vi "my diraction.vi"(7 "?":T2[](array[typedef]), 8 "Empty Directions":T1[](array[typedef]), 9 "my diraction":T1, 10 "curve_rate":dbl) -> (0 "you may act":bool, 1 "Direction for act":i16, 3 "Direction":T1)   [LabVIEW 2020, in "The_Hill_Youth.lvlib" / "MySquare.lvclass"]
uses:
  MySquare.lvclass
  SquareBattle/Direction.ctl
  MyTeam/map_point.ctl
  SquareBattle/SquareBattle.lvlib
panel:
  out "32bit integer":i32
  out "Waveform Chart":dbl(graph)
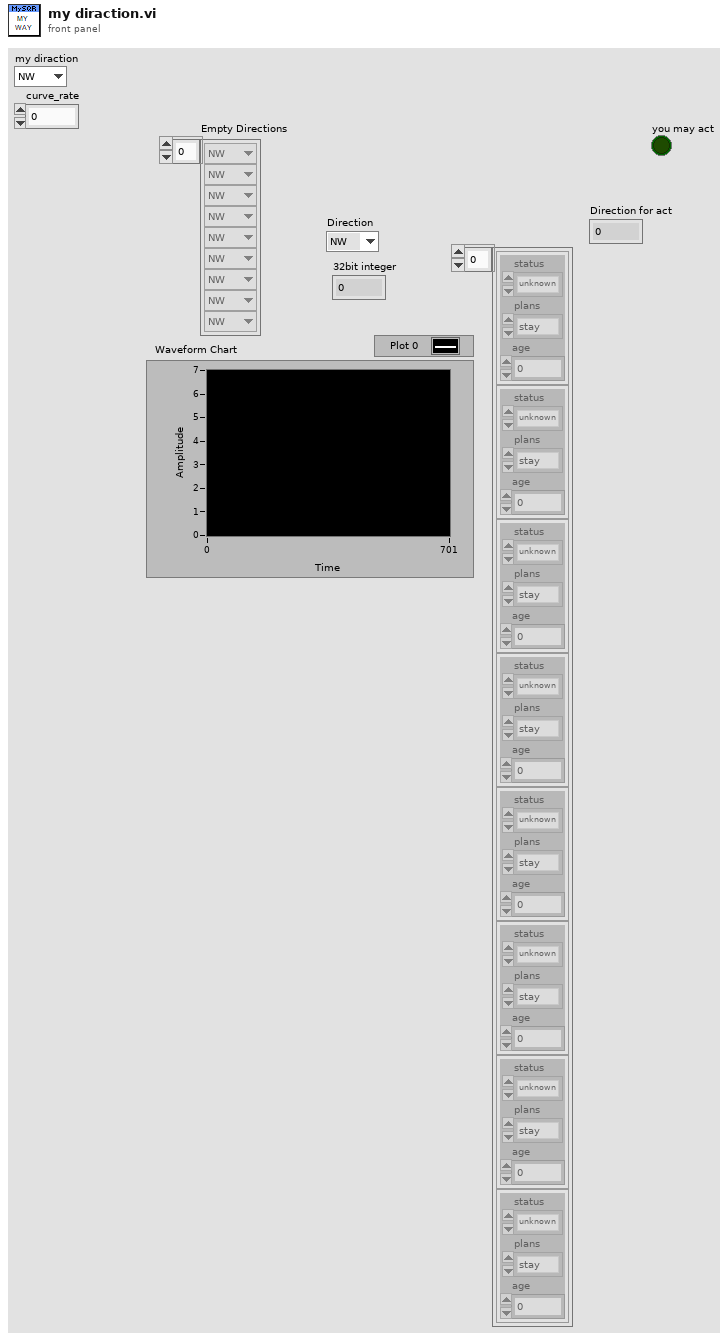
[diagram p1: front panel]
types:
  T1 = typedef "SquareBattle.lvlib/Direction.ctl" = enum16{"NW", "N", "NE", "E", "SE", "S", "SW", "W"}
  T2 = typedef "map_point.ctl" = cluster{"status":enum16{"unknown", "frind", "enemy", "empty"}, "plans":enum16{"stay", "duplicate", "attack", "move to", "no plans"}, "age":dbl}
  T3 = enum16{"stay", "duplicate", "attack", "move to", "no plans"}
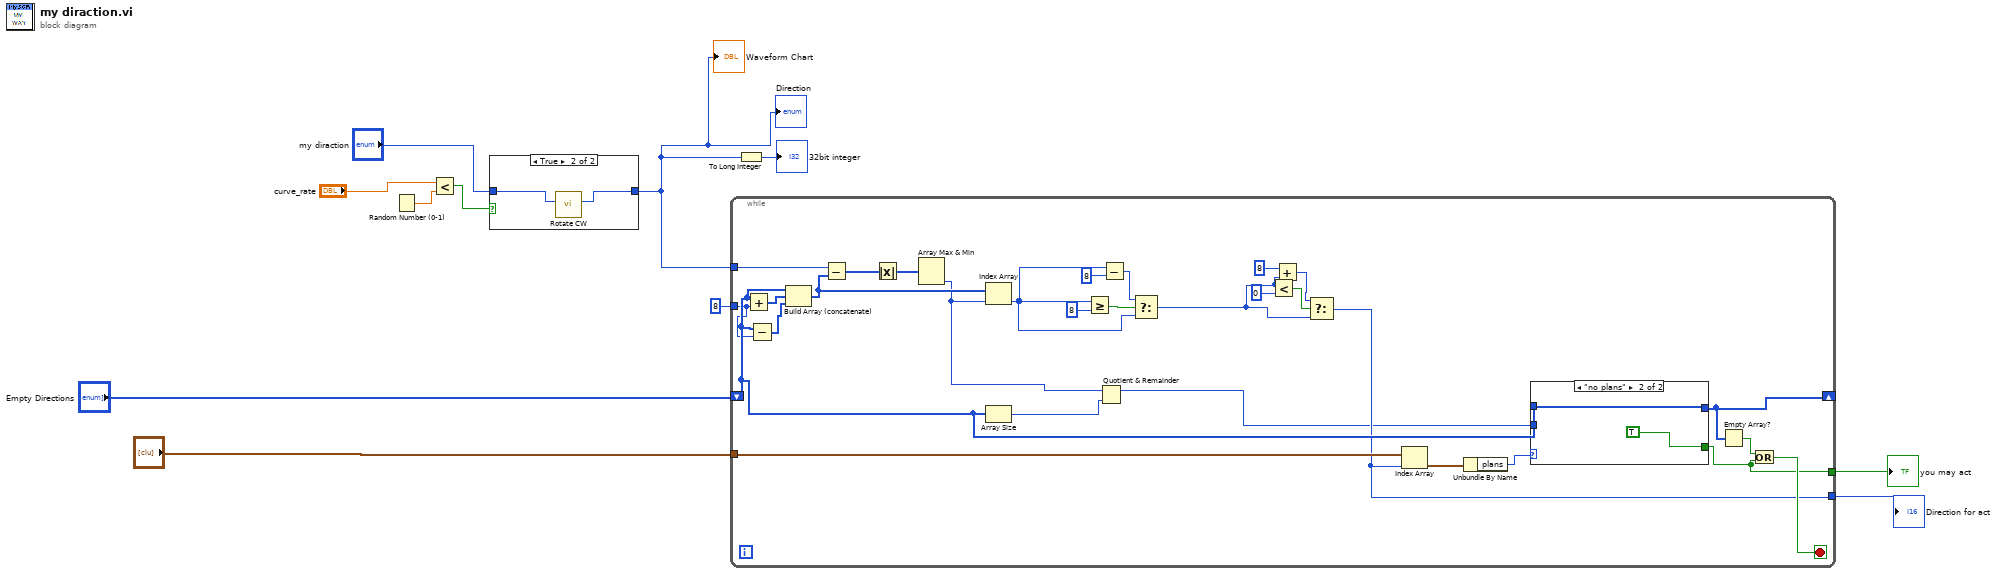
[diagram p0: block diagram]
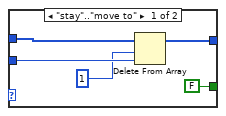
[diagram p3: hidden frame]
diagram:
  n1 = Random Number (0-1)() -> (number: 0 to 1=w5:dbl)
  n2 = Less?(x="curve_rate", y=w5) -> (x < y?=w4:bool)
  n3 = case shown="True" w4 {
    tunnel: "my diraction" -> [w12 w14]
    tunnel: [w12 w13] -> w2
    frame False {
    }
    frame True {
      n4 = call "Rotate CW.vi"("Direction"=w14) -> ("CW Rotated"=w13:T1)  [unwired: 10 in]
    }
  }
  "Direction" <- w2
  "Waveform Chart" <- w2
  n5 = while {
    tunnel: "?" -> [w43]
    tunnel: 8 -> [w25]
    tunnel: w2 -> [w41]
    shift-right: [w31] -> _
    shift-left: "Empty Directions" -> [w26]
    tunnel: [w23] -> w7
    tunnel: [w28] -> w8
    stop <- w29 stop-if-true
    n6 = Add(x=w26, y=w25) -> (x+y=w39:i32[])
    n7 = Subtract(x=w26, y=w25) -> (x-y=w24:i32[])
    n8 = Build Array (concatenate)(w26, w39, w24) -> (w37:i32[])
    n9 = Subtract(x=w41, y=w37) -> (x-y=w40:i32[])
    n10 = Absolute Value(x=w40) -> (abs(x)=w38:i32[])
    n11 = Array Max & Min(array=w38) -> (min index (indices)=w16:i32)  [unwired: 3 out]
    n12 = Index Array(array=w37, index=w16) -> (element=w32:i32)
    n13 = Array Size(array=w26) -> (size(s)=w17:i32)
    n14 = Greater Or Equal?(x=w32, y=8) -> (x >= y?=w33:bool)
    n15 = Quotient & Remainder(x=w16, y=w17) -> (x-y*floor(x/y)=w15:i32)  [unwired: 1 out]
    n16 = Subtract(x=w32, y=8) -> (x-y=w34:i32)
    n17 = Select(t=w34, s=w33, f=w32) -> (s? t:f=w20:i32)
    n18 = Less?(x=w20, y=0) -> (x < y?=w21:bool)
    n19 = Add(x=8, y=w20) -> (x+y=w18:i32)
    n20 = Select(t=w18, s=w21, f=w20) -> (s? t:f=w23:i32)
    n21 = Index Array(array=w43, index=w23) -> (element=w42:T2)
    n22 = Unbundle By Name(w42) -> ("plans"=w27:T3)
    n23 = case shown="\"no plans\"" w27 {
      tunnel: [FALSE TRUE] -> w28
      tunnel: w15 -> [w47 _]
      tunnel: w26 -> [w45 w49]
      tunnel: [w44 w49] -> w31
      frame "stay".."move to" {
        n24 = Delete From Array(array=w45, length=1, index=w47) -> (array with subset deleted=w44:T1[])  [unwired: 1 out]
      }
      frame "no plans" {
      }
    }
    n25 = Empty Array?(array=w31) -> (empty?=w30:bool)
    n26 = Or(x=w30, y=w28) -> (x .or. y?=w29:bool)
  }
  "you may act" <- w8
  "Direction for act" <- w7
  n27 = To Long Integer(number=w2) -> (32bit integer=→"32bit integer":i32)
